vi "Optionen_Setzen.vi"(8 "error in (no error)":errorcluster caption="Fehler (Eingang, kein Fehler)", 10 "Optionen (Eingang)":T1, 11 "Optionen Anzeige (Eingang)":refnum<vi>) -> (0 "error out":errorcluster caption="Fehler (Ausgang)")   [LabVIEW 2020, in "System Einstellungen V2.lvlib"]
uses:
  System Einstellungen V2.lvlib
  Optionen.ctl
  <vilib>/Utility/Data Type/NI_Data Type.lvlib
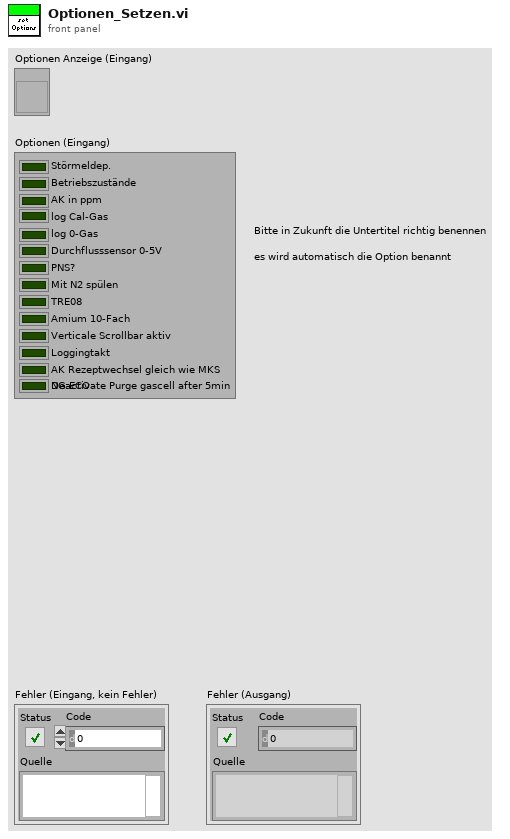
[diagram p1: front panel]
types:
  T1 = typedef "System Einstellungen V2.lvlib/Optionen.ctl" = cluster{"Störmeldep.":bool, "Betriebszustände":bool, "AK in ppm":bool, "log Cal-Gas":bool, "log 0-Gas":bool, "Durchflusssensor 0-5V":bool, "PNS?":bool, "Mit N2 spülen":bool, "TRE08":bool, "Amium 10-Fach":bool, "Verticale Scrollbar aktiv":bool, "Loggingtakt":bool, "AK Rezeptwechsel gleich wie MKS":bool, "NG ECO":bool}
  T2 = typedef "NI_Data Type.lvlib/Data Type.ctl" = enum8{"Invalid Type", "Void", "I8", "I16", "I32", "I64", "U8", "U16", "U32", "U64", "Single Float", "Double Float", "Extended Float", "Single Complex", "Double Complex", "Extended Complex", "Enum U8", "Enum U16", "Enum U32", "Enum U64", "Single Float With Unit", "Double Float With Unit", "Extended Float With Unit", "Single Complex with Unit", "Double Complex with Unit", "Extended Complex with Unit", "Boolean", "String", "Path", "Picture", "Tag", "Array", "Cluster", "Variant", "LV Variant", "Waveform", "Timestamp", "Digital Waveform", "Digital Data", "ExpressData", "Refnum", "External Data", "VI", "Poly VI", "LabVIEW Class Instance", "Fixed Point", "Set Collection", "Map Collection"}
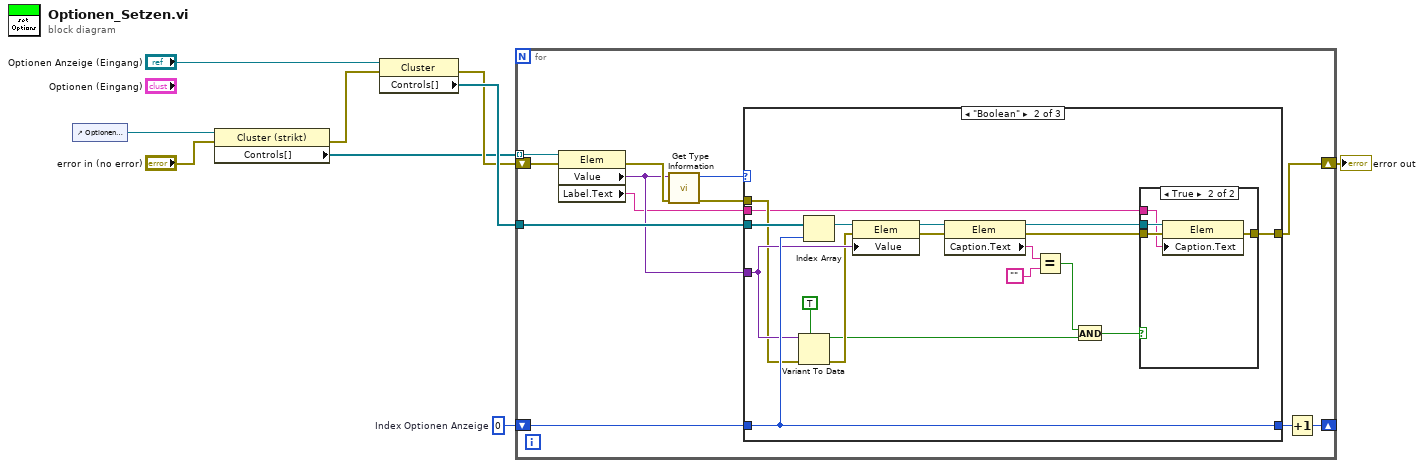
[diagram p0: block diagram]
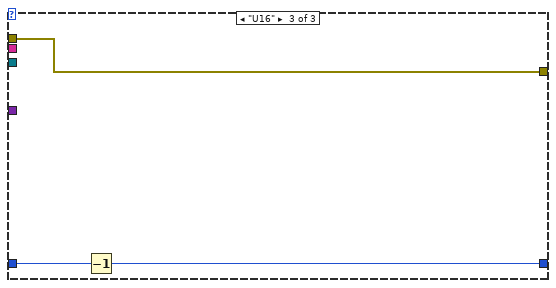
[diagram p4: hidden frame]
diagram:
  w2 = 0  # Index Optionen Anzeige
  n1 = control-ref of="Optionen (Eingang)"() -> (w5:refnum<vi>)
  n2 = property class="Cluster (strikt)"(reference=w5, error in="error in (no error)") -> (error out=w3:errorcluster, "Controls[]"=w1:refnum<vi>[])  [unwired: 1 out]
  n3 = property class="Cluster"(reference="Optionen Anzeige (Eingang)", error in=w3) -> (error out=w7:errorcluster, "Controls[]"=w8:refnum<vi>[])  [unwired: 1 out]
  n4 = for {
    tunnel: w8 -> [w21]
    shift-right: [w20] -> w6
    shift-left: w7 -> [w18]
    shift-right: [w13] -> _
    shift-left: w2 -> [w15]
    tunnel: w1 -> [w17] mode=indexing
    n5 = property class="Elem"(reference=w17, error in=w18) -> (error out=w19:errorcluster, "Value"=w12:variant, "Label.Text"=w10:string)  [unwired: 1 out]
    n6 = call <vilib>:"Get Type Information.vi"("error in (no error)"=w19, "variant"=w12) -> ("error out"=w11:errorcluster, "type"=w16:T2)  [unwired: 5 in, 3 out]
    n7 = case shown="\"Boolean\"" w16 {
      tunnel: w21 -> [_ w41 _]
      tunnel: [w22 w26 w47] -> w20
      tunnel: w15 -> [w23 w39 w49]
      tunnel: [w23 w39 w48] -> w14
      tunnel: w12 -> [_ w33 _]
      tunnel: w11 -> [w22 w32 w47]
      tunnel: w10 -> [_ w24 _]
      frame "Invalid Type", Default {
      }
      frame "Boolean" {
        n8 = Variant To Data(error in=w32, type=TRUE, Variant=w33) -> (data=w29:bool, error out=w31:errorcluster)
        n9 = Index Array(array=w41, index=w39) -> (element=w40:refnum<vi>)
        n10 = property class="Elem"(reference=w40, error in=w31, "Value"=w33) -> (reference out=w37:refnum<vi>, error out=w36:errorcluster)
        n11 = property class="Elem"(reference=w37, error in=w36) -> (reference out=w28:refnum<vi>, error out=w27:errorcluster, "Caption.Text"=w35:string)
        n12 = Equal?(x=w35, y="") -> (x = y?=w30:bool)
        n13 = And(x=w30, y=w29) -> (x .and. y?=w25:bool)
        n14 = case shown="True" w25 {
          tunnel: w28 -> [_ w46]
          tunnel: w27 -> [w42 w45]
          tunnel: [w42 w44] -> w26
          tunnel: w24 -> [_ w43]
          frame False {
          }
          frame True {
            n15 = property class="Elem"(reference=w46, error in=w45, "Caption.Text"=w43) -> (error out=w44:errorcluster)  [unwired: 1 out]
          }
        }
      }
      frame "U16" {
        n16 = Decrement(x=w49) -> (x-1=w48:i32)
      }
    }
    n17 = Increment(x=w14) -> (x+1=w13:i32)
  }
  "error out" <- w6
